vi "test - 单串口.vi"() -> ()   [LabVIEW 2017]
uses:
  <vilib>/Platform/TimedLoop/XDataNode/timing_clust.ctl
  <vilib>/Platform/TimedLoop/XDataNode/nitl_modes.ctl
  <vilib>/Platform/TimedLoop/XDataNode/wakeup.ctl
  <vilib>/Instr/_visa.llb/VISA Configure Serial Port (Instr).vi
  <vilib>/Platform/TimedLoop/XDataNode/XDataNode.xnode
  <vilib>/Platform/TimedLoop/XDataNode/XDNodeRunTimeDep.lvlib
panel:
  in  "停止":bool
  out "返回数 2":u32
  out "读取缓冲区1":string="i"
  in  "输出串口（com13）":refnum<visa-resource-name>="COM13"
  in  "输入串口（com11）":refnum<visa-resource-name>="COM11"
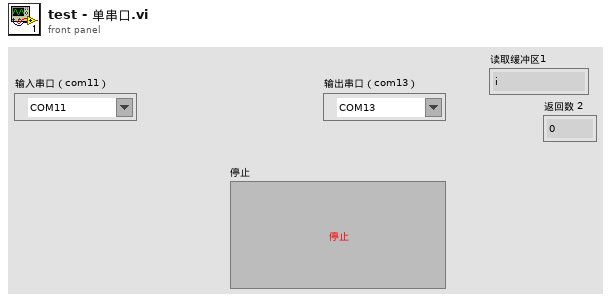
[diagram p1: front panel]
types:
  T1 = typedef "XDNodeRunTimeDep.lvlib/timing_clust.ctl" = cluster{"Expected End [f-1]":u64, "Actual End [f-1]":u64, "Finished Late? [f-1]":bool, "Expected End [i-1]":u64, "Actual End [i-1]":u64, "Finished Late? [i-1]":bool, "Expected Start [i]":u64, "Actual Start [i]":u64, "Expected Start [f]":u64, "Actual Start [f]":u64, "Source Name":string, "Structure Name":string, "Period":i64, "Deadline":i64, "Offset":i64, "Start":i64, "Priority":i32, "Timeout":i32, "Mode":T2, "Wakeup Reason":T3, "Error":errorcluster, "Source Type":string, "Secondary Source Type":string, "Global End Time":u64, "Global Start Time":u64, "Frame Duration":u64, "Iteration Duration":u64, "Assigned CPU":i32, "I/O Scan Engine Mode":u32}
  T2 = typedef "XDNodeRunTimeDep.lvlib/nitl_modes.ctl" = enum32{"No Change", "Process missed periods, maintain original phase", "Discard missed periods, maintain original phase", "Process missed periods, ignore original phase", "Discard missed periods, ignore original phase"}
  T3 = typedef "XDNodeRunTimeDep.lvlib/wakeup.ctl" = enum32{"Normal", "Aborted", "Asynchronous wakeup", "Timing source error", "Timed loop error", "Timeout"}
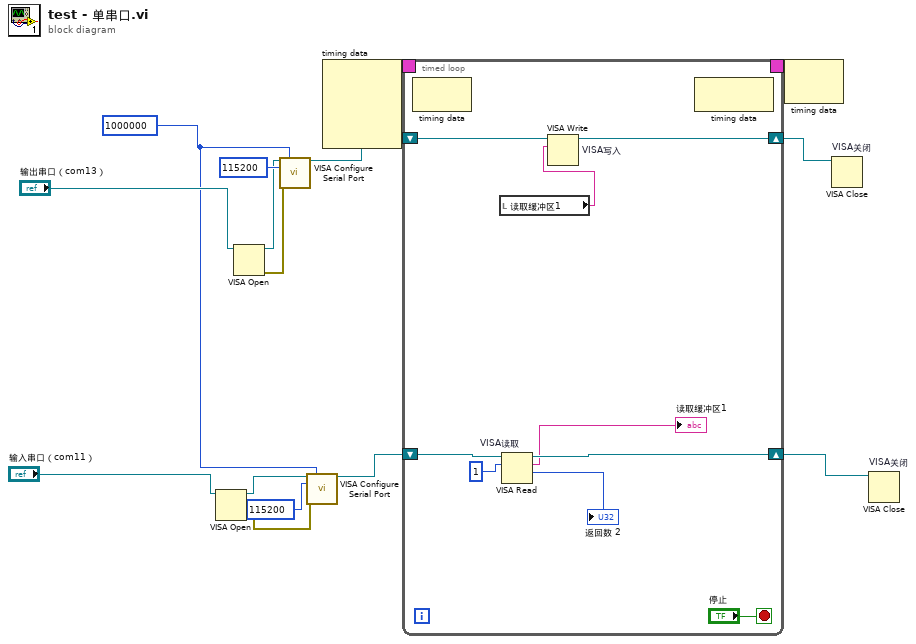
[diagram p0: block diagram]
diagram:
  w1 = u32 1000000 ("timeout (10sec)")
  n1 = VISA Open(VISA resource name="输入串口（com11）") -> (VISA resource name=w2:refnum<visa-resource-name>, error out=w4:errorcluster)  [unwired: 4 in]
  n2 = VISA Open(VISA resource name="输出串口（com13）") -> (VISA resource name=w5:refnum<visa-resource-name>, error out=w7:errorcluster)  [unwired: 4 in]
  n3 = call-poly "VISA Configure Serial Port"("VISA resource name"=w5, "timeout (10sec)"=w1, "baud rate (9600)"=u32 115200, "error in (no error)"=w7) -> ("VISA resource name out"=w12:refnum<visa-resource-name>)  [unwired: 10 in, 1 out]
  n4 = call-poly "VISA Configure Serial Port"("VISA resource name"=w2, "timeout (10sec)"=w1, "baud rate (9600)"=u32 115200, "error in (no error)"=w4) -> ("VISA resource name out"=w14:refnum<visa-resource-name>)  [unwired: 10 in, 1 out]
  n5 = node-c288() -> (w9:T1)  [unwired: 4 in]
  n6 = timed-loop {
    timing: w9 -> [_]
    timing-out: [_] -> w8
    shift-right: [w22] -> w11
    shift-left: w14 -> [w24]
    shift-right: [w21] -> w10
    shift-left: w12 -> [w23]
    stop <- "停止" stop-if-true
    n7 = node-c288() -> ()  [unwired: 1 in, 1 out]
    n8 = local read "读取缓冲区1"() -> (w20:string)
    n9 = VISA Read "VISA读取"(VISA resource name=w24, byte count=u32 1 ("字节总数")) -> (VISA resource name out=w22:refnum<visa-resource-name>, read buffer=→"读取缓冲区1":string, return count=→"返回数 2":u32)  [unwired: 1 in, 1 out]
    n10 = VISA Write "VISA写入"(VISA resource name=w23, write buffer=w20) -> (VISA resource name out=w21:refnum<visa-resource-name>)  [unwired: 1 in, 2 out]
    n11 = node-c288() -> ()  [unwired: 1 in, 1 out]
  }
  n12 = node-c288(w8) -> ()  [unwired: 1 out]
  n13 = VISA Close "VISA关闭"(VISA resource name=w10) -> ()  [unwired: 1 in, 1 out]
  n14 = VISA Close "VISA关闭"(VISA resource name=w11) -> ()  [unwired: 1 in, 1 out]
